vi "SCARA Inverse Kinematics.vi"(8 "error in (no error)":errorcluster, 10 "end effector position":dbl[](array[numeric]), 11 "SCARA serial arm in":refnum<class "NI_Robotics_SCARA Serial Arm Class.lvclass">) -> (0 "error out":errorcluster, 2 "joint positions":dbl[][](array[numeric]), 3 "SCARA serial arm out":refnum<class "NI_Robotics_SCARA Serial Arm Class.lvclass">)   [LabVIEW 2017, in "NI_Robotics_SCARA Serial Arm Class.lvclass"]
doc: "Returns the joint angles of a 6R, 5R, or SCARA arm given the posture of the end effector relative to the arm base. Wire data to the <B>X</B><B>_serial arm in</B> input, where <B>X</B> is the arm type, to determine the polymorphic instance to use or manually select the instance."
uses:
  <vilib>/robotics/Kinematics/Analytical/SCARA/NI_Robotics_SCARA Serial Arm Class.lvclass
  <vilib>/robotics/Kinematics/Analytical/SCARA/NI_Robotics_SCARA Serial Arm Class.lvclass/NI_Robotics_SCARA Serial Arm Class.ctl
  <vilib>/robotics/Utilities/NI_Robotics Utilities.lvlib
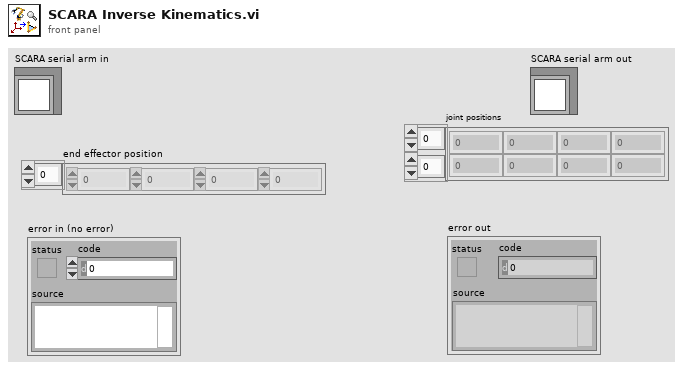
[diagram p1: front panel]
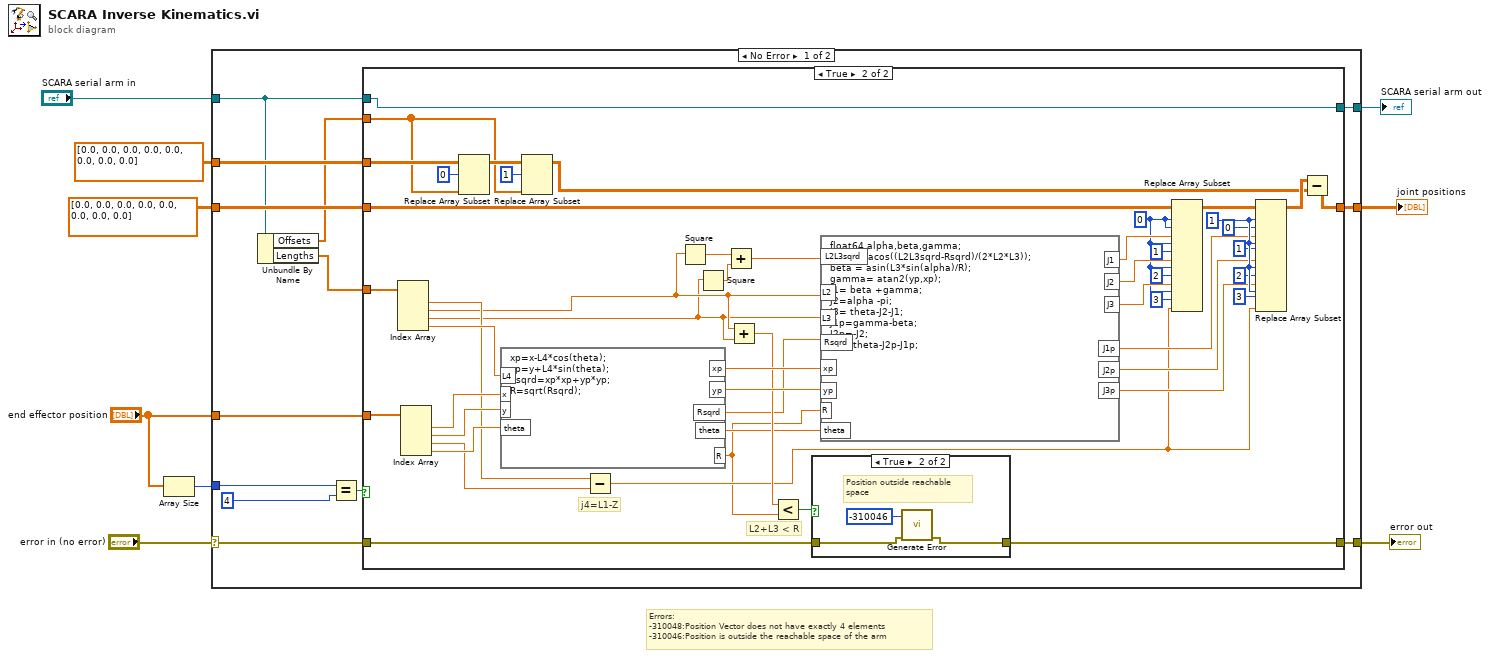
[diagram p0: block diagram]
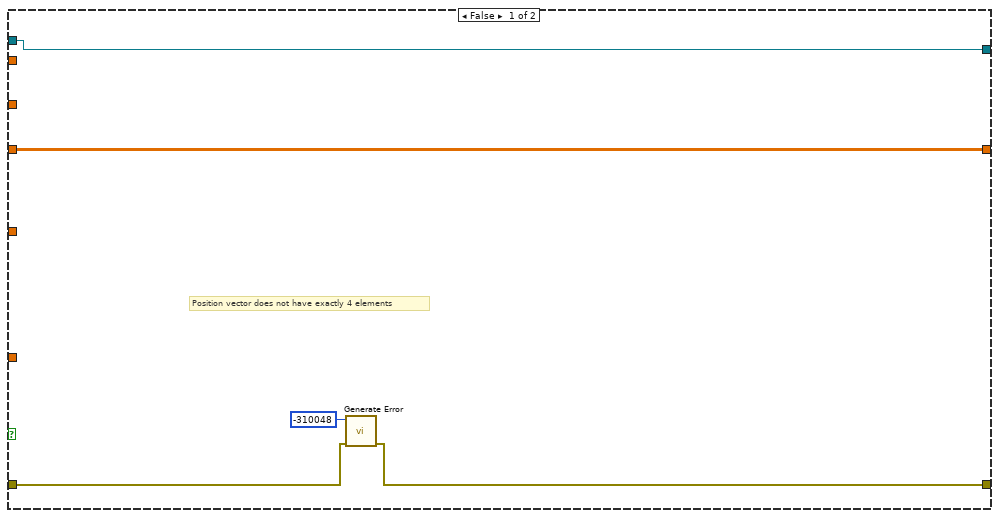
[diagram p2: hidden frame]
diagram:
  # "Errors:\n-310048:Position Vector does not have exactly 4 elements\n-310046:Position is outside the reachable space of the arm"
  n1 = Array Size(array="end effector position") -> (size(s)=w7:i32)
  n2 = case shown="No Error" "error in (no error)" {
    selector: "error in (no error)" -> [w19 w83]
    tunnel: [w18 w83] -> w8
    tunnel: w7 -> [w21 _]
    tunnel: "end effector position" -> [w17 _]
    tunnel: [w16 w82] -> w4
    tunnel: dbl[][] [[0.0, 0.0, 0.0, 0.0], [0.0, 0.0, 0.0, 0.0]] -> [w15 w82]
    tunnel: dbl[][] [[0.0, 0.0, 0.0, 0.0], [0.0, 0.0, 0.0, 0.0]] -> [w14 _]
    tunnel: "SCARA serial arm in" -> [w13 w81]
    tunnel: [w10 w81] -> w1
    frame No Error {
      n3 = Unbundle By Name(w13) -> ("Offsets"=w12:dbl[], "Lengths"=w11:dbl[])
      n4 = Equal?(x=w21, y=4) -> (x = y?=w22:bool)
      n5 = case shown="True" w22 {
        tunnel: w19 -> [w26 w69]
        tunnel: [w25 w68] -> w18
        tunnel: w11 -> [_ w76]
        tunnel: w12 -> [_ w35]
        tunnel: w17 -> [_ w75]
        tunnel: [w24 w32] -> w16
        tunnel: w15 -> [w24 w59]
        tunnel: w14 -> [_ w39]
        tunnel: w13 -> [w23 w31]
        tunnel: [w23 w31] -> w10
        frame False {
          # "Position vector does not have exactly 4 elements"
          n6 = call <vilib>:"Generate Error.vi"("error in (no error)"=w26, "code"=-310048) -> ("error out"=w25:errorcluster)  [unwired: 9 in]
        }
        frame True {
          w47 = 1 ("index (row)")
          w52 = 0 ("index (row)")
          # "j4=L1-Z"
          # "L2+L3 < R"
          n7 = Index Array(array=w76) -> (element #1=w64:dbl, element #2=w56:dbl, element #3=w55:dbl, element #4=w74:dbl)  [unwired: 4 in]
          n8 = Index Array(array=w75) -> (element #1=w73:dbl, element #2=w72:dbl, element #3=w63:dbl, element #4=w71:dbl)  [unwired: 4 in]
          n9 = Replace Array Subset(array=w39, new element=w35, index (row)=0) -> (w37:dbl[][])  [unwired: 1 in]
          n10 = formula code="xp=x-L4*cos(theta);\nyp=y+L4*sin(theta);\nRsqrd=xp*xp+yp*yp;\nR=sqrt(Rsqrd);"("L4"=w74, "x"=w73, "y"=w72, "theta"=w71) -> ("xp"=w66:dbl, "yp"=w65:dbl, "Rsqrd"=w30:dbl, "theta"=w53:dbl, "R"=w29:dbl)
          n11 = Replace Array Subset(array=w37, new element=w35, index (row)=1) -> (w33:dbl[][])  [unwired: 1 in]
          n12 = Subtract(x=w64, y=w63) -> (x-y=w40:dbl)
          n13 = Square(x=w56) -> (x^2=w58:dbl)
          n14 = Square(x=w55) -> (x^2=w57:dbl)
          n15 = Add(x=w58, y=w57) -> (x+y=w67:dbl)
          n16 = Add(x=w56, y=w55) -> (x+y=w54:dbl)
          n17 = Less?(x=w54, y=w29) -> (x < y?=w70:bool)
          n18 = case shown="True" w70 {
            tunnel: w69 -> [w77 w80]
            tunnel: [w77 w79] -> w68
            frame False {
            }
            frame True {
              # "Position outside reachable\nspace"
              n19 = call <vilib>:"Generate Error.vi"("error in (no error)"=w80, "code"=-310046) -> ("error out"=w79:errorcluster)  [unwired: 9 in]
            }
          }
          n20 = formula code="float64 alpha,beta,gamma;\nalpha= acos((L2L3sqrd-Rsqrd)/(2*L2*L3));\nbeta = asin(L3*sin(alpha)/R);\ngamma= atan2(yp,xp);\nJ1= beta +gamma;\nJ2=alpha -pi;\nJ3= theta-J2-J1;\nJ1p=gamma-beta;\nJ2p=-J2;\nJ3p=theta-J2p-J1p;"("L2L3sqrd"=w67, "L2"=w56, "L3"=w55, "Rsqrd"=w30, "xp"=w66, "yp"=w65, "theta"=w53, "R"=w29) -> ("J1"=w62:dbl, "J2"=w61:dbl, "J3"=w60:dbl, "J1p"=w43:dbl, "J2p"=w42:dbl, "J3p"=w41:dbl)
          n21 = Replace Array Subset(array=w59, new element #1=w62, index (row) #1=w52, index (col) #1=w52, new element #2=w61, index (row) #2=w52, index (col) #2=1 ("disabled index (col)"), new element #3=w60, index (row) #3=w52, index (col) #3=2 ("disabled index (col)"), new element #4=w40, index (row) #4=w52, index (col) #4=3 ("disabled index (col)")) -> (w48:dbl[][])
          n22 = Replace Array Subset(array=w48, new element #1=w43, index (row) #1=w47, index (col) #1=0 ("index (row)"), new element #2=w42, index (row) #2=w47, index (col) #2=1 ("disabled index (col)"), new element #3=w41, index (row) #3=w47, index (col) #3=2 ("disabled index (col)"), new element #4=w40, index (row) #4=w47, index (col) #4=3 ("disabled index (col)")) -> (w34:dbl[][])
          n23 = Subtract(x=w34, y=w33) -> (x-y=w32:dbl[][])
        }
      }
    }
    frame Error {
    }
  }
  "error out" <- w8
  "joint positions" <- w4
  "SCARA serial arm out" <- w1
